vi "actuate_singleJumpExp_v0.04.vi"(0 "Phase Cluster":T2, 1 "valve Time Cluster":T1, 2 "Didn't Lift?":bool, 3 "data in":T3={"daq_ao 1"="Dev1/ao0", "daq_ai 1"="Dev1/ai0", "experiment day folder"=path "D:/DATA/8-27-15 save func testing/test.lvm", "Multiclamp init error"=0, "Multiclamp Handle Out"=0, "sampling rate (Hz)"=10000, "trial name"=""}, 5 "PhaseLetter":string, 7 "controls array in":refnum<vi>[](array[refnum]), 9 "time to wait for solution change (min)":dbl=2.5 min=0.0 step=0.01, 11 "error in":errorcluster, 12 "common cluster":T6, 13 "individual controls in":T5) -> (4 "output cluster":T4={"daq_ao 2"="", "Duration (s)"=0.0, "Sample Freq (Hz)"=0.0, "Phase"=0.0, "Duty Cycle"=0.0, "Jump Filter Freq (Hz)"=0.0, "Number of Replicates"=1} {"Number of Replicates" min=1 max=10}, 6 "protocol waveform":waveform(dbl)(graph), 8 "jumptestMonitor":waveform(dbl)[](graph) caption="protocol response", 10 "control array out":refnum<vi>[](array[refnum]), 14 "experiment VI ref":refnum<vi>, 15 "error out":errorcluster)   [LabVIEW 2019]
uses:
  pipette cleaning/pressure box/cleaning_soft/controls/actuator_type.ctl
  pipette cleaning/pressure box/cleaning_soft/controls/actuator_cluster.ctl
  machine_vision/coordinate model vis/transform_properties_actuators.ctl
  machine_vision/controls/transform_cluster_actuator.ctl
  controls/NH_method.ctl
  pipette cleaning/pressure box/cleaning_soft/controls/pressure_box_type.ctl
  pipette cleaning/pressure box/cleaning_soft/controls/pressure_box_control.ctl
  multipatch/controls/multipatch_common_controls_v4.ctl
  controls/memtest_def.ctl
  multipatch/controls/multipatch_individual_controls_v5.ctl
  Controls/Data.ctl
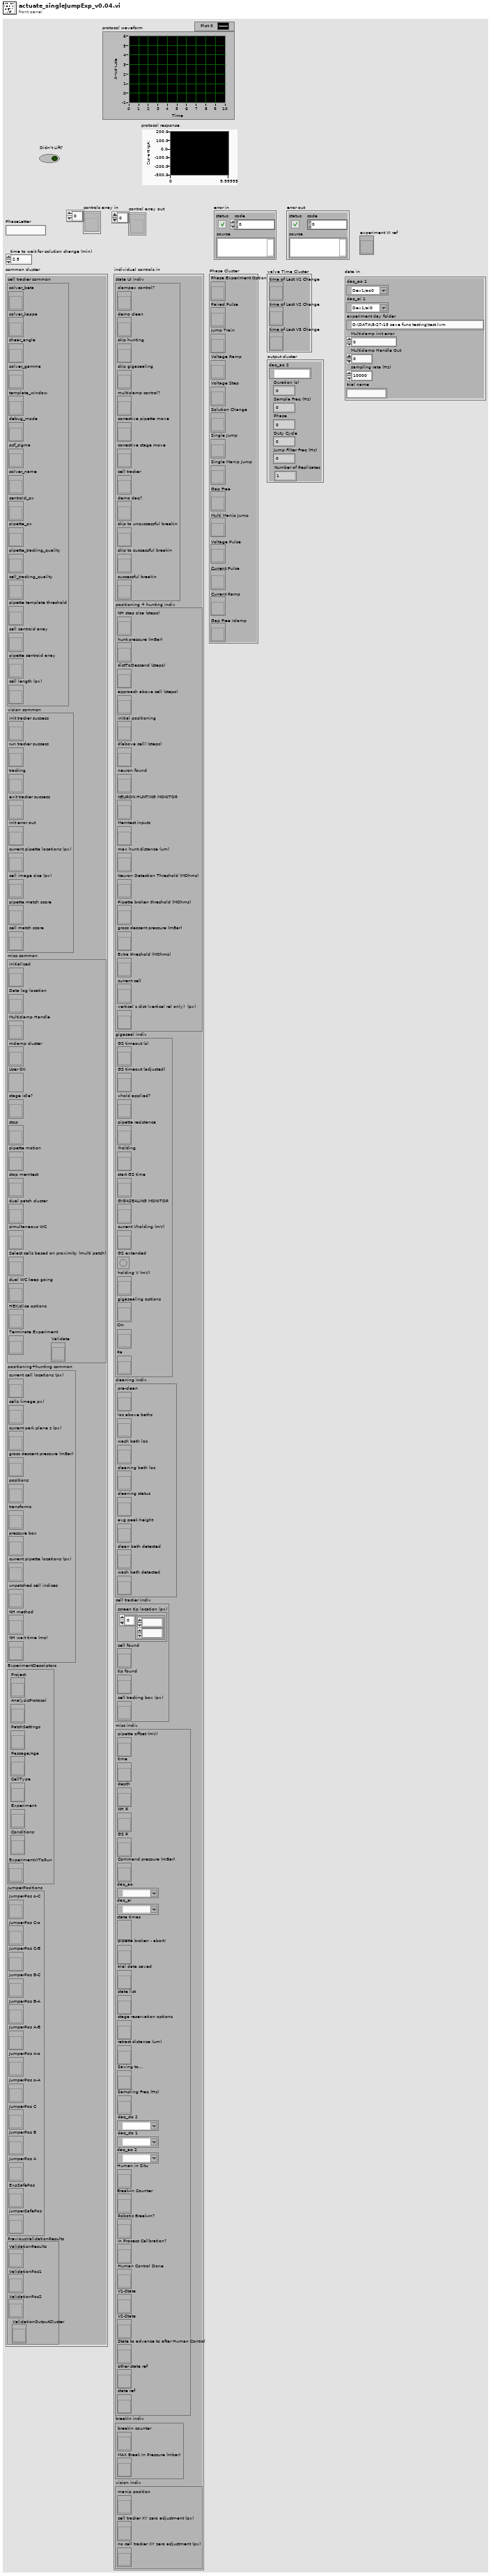
[diagram p1: front panel]
types:
  T1 = cluster{"time of Last V1 Change":refnum<vi>, "time of Last V2 Change":refnum<vi>, "time of Last V3 Change":refnum<vi>}
  T2 = cluster{"Phase Experiment Option":refnum<vi>, "Paired Pulse":refnum<vi>, "Jump Train":refnum<vi>, "Voltage Ramp":refnum<vi>, "Voltage Step":refnum<vi>, "Solution Change":refnum<vi>, "Single Jump":refnum<vi>, "Single Manip Jump":refnum<vi>, "Gap Free":refnum<vi>, "Multi Manip Jump":refnum<vi>, "Voltage Pulse":refnum<vi>, "Current Pulse":refnum<vi>, "Current Ramp":refnum<vi>, "Gap Free Iclamp":refnum<vi>}
  T3 = typedef "Data.ctl" = cluster{"daq_ao 1":tag, "daq_ai 1":tag, "experiment day folder":path, "Multiclamp init error":i32, "Multiclamp Handle Out":u32, "sampling rate (Hz)":i32, "trial name":string}
  T4 = cluster{"daq_ao 2":tag, "Duration (s)":dbl, "Sample Freq (Hz)":dbl, "Phase":dbl, "Duty Cycle":dbl, "Jump Filter Freq (Hz)":dbl, "Number of Replicates":i16}
  T5 = typedef "multipatch_individual_controls_v5.ctl" = cluster{"state UI indiv":cluster{"clampex control?":refnum<vi>, "demo clean":refnum<vi>, "skip hunting":refnum<vi>, "skip gigasealing":refnum<vi>, "multiclamp control?":refnum<vi>, "corrective pipette move":refnum<vi>, "corrective stage move":refnum<vi>, "cell tracker":refnum<vi>, "demo daq?":refnum<vi>, "skip to unsuccessful breakin":refnum<vi>, "skip to successful breakin":refnum<vi>, "successful breakin":refnum<vi>}, "positioning + hunting indiv":cluster{"NH step size (steps)":refnum<vi>, "hunt pressure (mBar)":refnum<vi>, "distToDescend (steps)":refnum<vi>, "approach above cell (steps)":refnum<vi>, "initial positioning":refnum<vi>, "d(above cell) (steps)":refnum<vi>, "neuron found":refnum<vi>, "NEURON HUNTING MONITOR":refnum<vi>, "Memtest inputs":refnum<vi>, "max hunt distance (um)":refnum<vi>, "Neuron Detection Threshold (MOhms)":refnum<vi>, "Pipette broken threshold (MOhms)":refnum<vi>, "gross descent pressure (mBar)":refnum<vi>, "Extra threshold (MOhms)":refnum<vi>, "current cell":refnum<vi>, "vertical z dist (vertical rel only)  (px)":refnum<vi>}, "gigaseal indiv":cluster{"GS timeout (s)":refnum<vi>, "GS timeout (adjusted)":refnum<vi>, "vhold applied?":refnum<vi>, "pipette resistance":refnum<vi>, "Iholding":refnum<vi>, "start GS time":refnum<vi>, "GIGASEALING MONITOR":refnum<vi>, "current Vholding (mV)":refnum<vi>, "GS extended":refnum<vi>, "holding V (mV)":refnum<vi>, "gigasealing options":refnum<vi>, "Cm":refnum<vi>, "Ra ":refnum<vi>}, "cleaning indiv":cluster{"pre-clean":refnum<vi>, "loc above baths":refnum<vi>, "wash bath loc":refnum<vi>, "cleaning bath loc":refnum<vi>, "cleaning status":refnum<vi>, "avg peak height":refnum<vi>, "clean bath detected":refnum<vi>, "wash bath detected":refnum<vi>}, "cell tracker indiv":cluster{"screen tip location (px)":refnum<vi>, "cell found":refnum<vi>, "tip found":refnum<vi>, "cell tracking box (px)":refnum<vi>}, "misc indiv":cluster{"pipette offset (mV)":refnum<vi>, "time":refnum<vi>, "depth":refnum<vi>, "NH R":refnum<vi>, "GS R":refnum<vi>, "Command pressure (mBar)":refnum<vi>, "daq_ao":tag, "daq_ai":tag, "state times":refnum<vi>, "pipette broken - abort!":refnum<vi>, "trial data saved":refnum<vi>, "state list":refnum<vi>, "stage reservation options":refnum<vi>, "retract distance (um)":refnum<vi>, "Saving to...":refnum<vi>, "Sampling Freq (Hz)":refnum<vi>, "daq_do 2":tag, "daq_do 1":tag, "daq_ao 2":tag, "Human in Situ":refnum<vi>, "Break-In Counter":refnum<vi>, "Robotic Break-In?":refnum<vi>, "In Process Calibration?":refnum<vi>, "Human Control Done":refnum<vi>, "V1-State":refnum<vi>, "V2-State":refnum<vi>, "State to advance to after Human Control":refnum<vi>, "other state ref":refnum<vi>, "state ref":refnum<vi>}, "breakin indiv":cluster{"breakin counter":refnum<vi>, "MAX Break In Pressure (mbar)":refnum<vi>}, "vision indiv":cluster{"manip position":refnum<vi>, "cell tracker XY zero adjustment (px)":refnum<vi>, "no cell tracker XY zero adjustment (px)":refnum<vi>}}
  T6 = typedef "multipatch_common_controls_v4.ctl" = cluster{"cell tracker common":cluster{"solver_beta":refnum<vi>, "solver_kappa":refnum<vi>, "shear_angle":refnum<vi>, "solver_gamma":refnum<vi>, "template_window":refnum<vi>, "debug_mode":refnum<vi>, "psf_sigma":refnum<vi>, "solver_name":refnum<vi>, "centroid_px":refnum<vi>, "pipette_px":refnum<vi>, "pipette_tracking_quality":refnum<vi>, "cell_tracking_quality":refnum<vi>, "pipette template threshold":refnum<vi>, "cell centroid array":refnum<vi>, "pipette centroid array":refnum<vi>, "cell length (px)":refnum<vi>}, "vision common":cluster{"init tracker success":refnum<vi>, "run tracker success":refnum<vi>, "tracking":refnum<vi>, "exit tracker success":refnum<vi>, "init error out":refnum<vi>, "current pipette locations (px)":refnum<vi>, "cell image size (px)":refnum<vi>, "pipette match score":refnum<vi>, "cell match score":refnum<vi>}, "misc common":cluster{"initialized":refnum<vi>, "Data log location":refnum<vi>, "Multiclamp Handle":refnum<vi>, "mclamp cluster":refnum<vi>, "User OK":refnum<vi>, "stage idle?":refnum<vi>, "stop":refnum<vi>, "pipette motion":refnum<vi>, "stop memtest":refnum<vi>, "dual patch cluster":refnum<vi>, "simultaneous WC":refnum<vi>, "Select cells based on proximity (multi patch)":refnum<vi>, "dual WC keep going":refnum<vi>, "HEK/slice options":refnum<vi>, "Terminate Experiment":refnum<vi>, "Validate":refnum<vi>}, "positioning+hunting common":cluster{"current cell locations (px)":refnum<vi>, "cells (image px)":refnum<vi>, "current park plane z (px)":refnum<vi>, "gross descent pressure (mBar)":refnum<vi>, "positions":refnum<vi>, "transforms":refnum<vi>, "pressure box":refnum<vi>, "current pipette locations (px)":refnum<vi>, "unpatched cell indices":refnum<vi>, "NH method":refnum<vi>, "NH wait time (ms)":refnum<vi>}, "ExperimentDescriptors":cluster{"Project":refnum<vi>, "AnalysisProtocol":refnum<vi>, "PatchSettings":refnum<vi>, "Passage/Age":refnum<vi>, "CellType":refnum<vi>, "Experiment":refnum<vi>, "Conditions":refnum<vi>, "ExperimentVIToRun":refnum<vi>}, "JumperPositions":cluster{"JumperPos o-C":refnum<vi>, "JumperPos C-o":refnum<vi>, "JumperPos C-B":refnum<vi>, "JumperPos B-C":refnum<vi>, "JumperPos B-A":refnum<vi>, "JumperPos A-B":refnum<vi>, "JumperPos A-o":refnum<vi>, "JumperPos o-A":refnum<vi>, "JumperPos C":refnum<vi>, "JumperPos B":refnum<vi>, "JumperPos A":refnum<vi>, "ExpSafePos":refnum<vi>, "jumperSafePos":refnum<vi>}, "PreviousValidationResults":cluster{"ValidationResults":refnum<vi>, "ValidationPos1":refnum<vi>, "ValidationPos2":refnum<vi>, "ValidationOutputCluster":refnum<vi>}}
  T7 = cluster{"Which Position to use for Experiment":enum16{"Jumper Safe Position", "Experiment Safe Position", "Jumper Position A", "Jumper Position B", "Jumper Position C", "Jumper Position o-A", "Jumper Position A-o", "Jumper Position A-B", "Jumper Position B-A", "Jumper Position B-C", "Jumper Position C-B", "Jumper Position C-o", "Jumper Position o-C", "Don't Move"}, "Start Position (N)":string, "Jump Position (m)":string, "Duration (s)":dbl, "Delay (s)":dbl, "Pulse Width (s)":dbl, "Valve 1 Position":i16, "Valve 2 Position":i16, "Replicates":dbl, "Vholding (mV)":dbl, "Valve 3 Position":i16, "valve 1 used now?":bool, "valve 2 used now?":bool, "valve 3 used now? ":bool, "protocol Preview":waveform(dbl)[]}
  T8 = enum16{"Jumper Safe Position", "Experiment Safe Position", "Jumper Position A", "Jumper Position B", "Jumper Position C", "Jumper Position o-A", "Jumper Position A-o", "Jumper Position A-B", "Jumper Position B-A", "Jumper Position B-C", "Jumper Position C-B", "Jumper Position C-o", "Jumper Position o-C", "Don't Move"}
  T9 = enum16{"manipulator 1", "manipulator 2", "manipulator 3", "manipulator 4"}
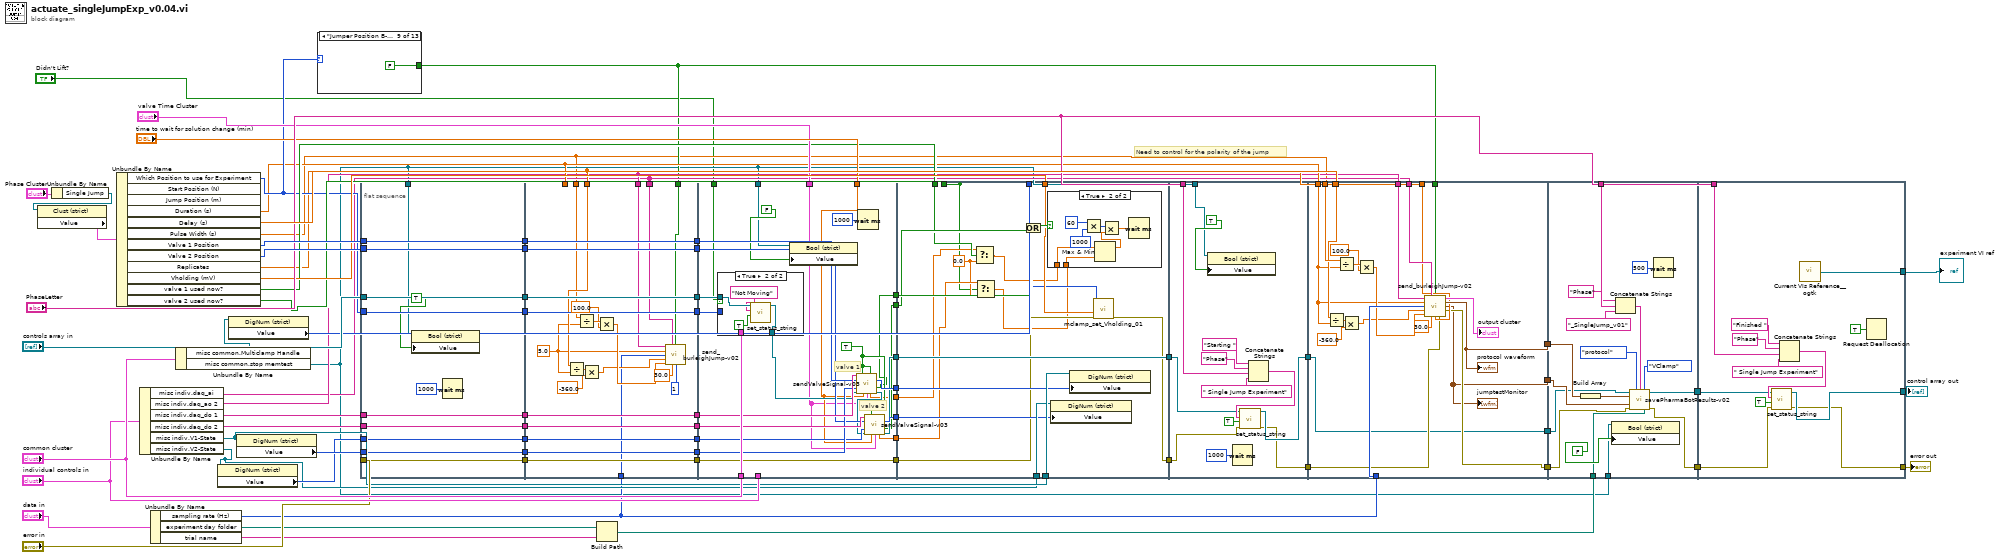
[diagram p0: block diagram]
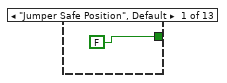
[diagram p2: hidden frame]
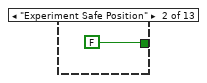
[diagram p3: hidden frame]
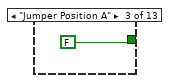
[diagram p4: hidden frame]
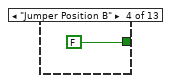
[diagram p5: hidden frame]
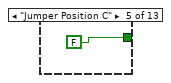
[diagram p6: hidden frame]
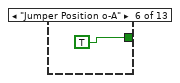
[diagram p7: hidden frame]
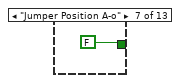
[diagram p8: hidden frame]
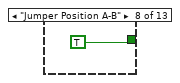
[diagram p9: hidden frame]
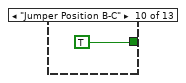
[diagram p10: hidden frame]
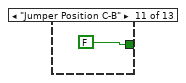
[diagram p11: hidden frame]
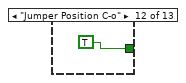
[diagram p12: hidden frame]
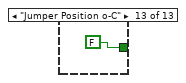
[diagram p13: hidden frame]
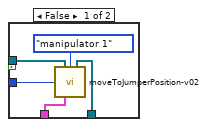
[diagram p14: hidden frame]
diagram:
  # "Need to control for the polarity of the jump"
  n1 = Unbundle By Name("Phase Cluster") -> ("Single Jump"=w55:refnum<vi>)
  n2 = property class="Clust (strict)"(reference=w55) -> ("Value"=w54:T7)  [unwired: 1 in, 2 out]
  n3 = Unbundle By Name(w54) -> ("Which Position to use for Experiment"=w29:T8, "Duration (s)"=w19:dbl, "Delay (s)"=w51:dbl, "Pulse Width (s)"=w3:dbl, "Valve 1 Position"=w53:i16, "Valve 2 Position"=w52:i16, "Replicates"=w18:dbl, "Vholding (mV)"=w38:dbl, "valve 1 used now?"=w31:bool, "valve 2 used now?"=w30:bool)  [unwired: 2 out]
  n4 = Unbundle By Name("individual controls in") -> ("misc indiv.daq_ai"=w15:tag, "misc indiv.daq_ao 2"=w16:tag, "misc indiv.daq_do 1"=w75:tag, "misc indiv.daq_do 2"=w74:tag, "misc indiv.V1-State"=w66:refnum<vi>, "misc indiv.V2-State"=w65:refnum<vi>)
  n5 = Unbundle By Name("data in") -> ("sampling rate (Hz)"=w17:i32, "experiment day folder"=w59:path, "trial name"=w58:string)
  n6 = Unbundle By Name("common cluster") -> ("misc common.Multiclamp Handle"=w37:refnum<vi>, "misc common.stop memtest"=w4:refnum<vi>)
  n7 = property class="DigNum (strict)"(reference=w65) -> ("Value"=w67:u16)  [unwired: 1 in, 2 out]
  n8 = property class="DigNum (strict)"(reference=w37) -> ("Value"=w36:u32)  [unwired: 1 in, 2 out]
  n9 = property class="DigNum (strict)"(reference=w66) -> ("Value"=w68:u16)  [unwired: 1 in, 2 out]
  n10 = case shown="\"Jumper Position B-A\"" w29 {
    tunnel: [FALSE FALSE FALSE FALSE FALSE TRUE FALSE TRUE FALSE TRUE FALSE TRUE FALSE] -> w14
    frame "Jumper Safe Position", Default {
    }
    frame "Experiment Safe Position" {
    }
    frame "Jumper Position A" {
    }
    frame "Jumper Position B" {
    }
    frame "Jumper Position C" {
    }
    frame "Jumper Position o-A" {
    }
    frame "Jumper Position A-o" {
    }
    frame "Jumper Position A-B" {
    }
    frame "Jumper Position B-A" {
    }
    frame "Jumper Position B-C" {
    }
    frame "Jumper Position C-B" {
    }
    frame "Jumper Position C-o" {
    }
    frame "Jumper Position o-C" {
    }
  }
  n11 = flat-sequence {
    tunnel: "controls array in" -> [w94]
    tunnel: w52 -> [w95]
    tunnel: w53 -> [w96]
    tunnel: w67 -> [w97]
    tunnel: w68 -> [w98]
    tunnel: "error in" -> [w99]
    tunnel: w74 -> [w100]
    tunnel: w75 -> [w101]
    tunnel: w29 -> [w102]
    tunnel: [w102] -> w13
    tunnel: [w101] -> w12
    tunnel: [w100] -> w11
    tunnel: [w99] -> w10
    tunnel: [w98] -> w9
    tunnel: [w97] -> w8
    tunnel: [w96] -> w7
    tunnel: [w95] -> w6
    tunnel: [w94] -> w5
    tunnel: w4 -> [w92]
    tunnel: [w126] -> w28
    tunnel: [w125] -> w27
    tunnel: [w124] -> w26
    tunnel: [w123] -> w25
    tunnel: [w122] -> w24
    tunnel: [w121] -> w23
    tunnel: [w120] -> w22
    tunnel: [w119] -> w21
    tunnel: [w118] -> w20
    tunnel: w19 -> [_]
    tunnel: w18 -> [w111]
    tunnel: w3 -> [w110]
    tunnel: w17 -> [w109]
    tunnel: w16 -> [w108]
    tunnel: w15 -> [w107]
    tunnel: w14 -> [w105]
    tunnel: w13 -> [w126]
    tunnel: w12 -> [w125]
    tunnel: w11 -> [w124]
    tunnel: w10 -> [w123]
    tunnel: w9 -> [w122]
    tunnel: w8 -> [w121]
    tunnel: w7 -> [w120]
    tunnel: w6 -> [w119]
    tunnel: w5 -> [w118]
    tunnel: "common cluster" -> [w151]
    tunnel: "individual controls in" -> [_]
    tunnel: [w148] -> w70
    tunnel: [w145] -> w64
    tunnel: [w144] -> w63
    tunnel: [w138] -> w45
    tunnel: [w136] -> w40
    tunnel: [w135] -> w39
    tunnel: "time to wait for solution change (min)" -> [w134]
    tunnel: "valve Time Cluster" -> [w133]
    tunnel: [w132] -> w33
    tunnel: [w131] -> w32
    tunnel: w28 -> [w152]
    tunnel: w27 -> [w150]
    tunnel: w26 -> [w149]
    tunnel: w25 -> [w148]
    tunnel: w24 -> [w147]
    tunnel: w23 -> [w146]
    tunnel: w22 -> [w143]
    tunnel: w21 -> [w142]
    tunnel: w20 -> [w141]
    tunnel: w4 -> [w129]
    tunnel: "Didn't Lift?" -> [w127]
    tunnel: [w169] -> w71
    tunnel: w70 -> [w171]
    tunnel: w66 -> [w180]
    tunnel: w65 -> [w179]
    tunnel: w64 -> [w178]
    tunnel: w63 -> [w177]
    tunnel: [w176] -> w46
    tunnel: w45 -> [w176]
    tunnel: w40 -> [w174]
    tunnel: w39 -> [w173]
    tunnel: w38 -> [w172]
    tunnel: w36 -> [w170]
    tunnel: w33 -> [w166]
    tunnel: w32 -> [w165]
    tunnel: w31 -> [w167]
    tunnel: [w162] -> _
    tunnel: w30 -> [w162]
    tunnel: w4 -> [w188]
    tunnel: [w190] -> w72
    tunnel: w71 -> [w191]
    tunnel: [w192] -> w47
    tunnel: w46 -> [w193]
    tunnel: "PhaseLetter" -> [w194]
    tunnel: w15 -> [w220]
    tunnel: w16 -> [w219]
    tunnel: w72 -> [w205]
    tunnel: [w217] -> w62
    tunnel: [w202] -> w61
    tunnel: w18 -> [w207]
    tunnel: w19 -> [w206]
    tunnel: w17 -> [w216]
    tunnel: w3 -> [w214]
    tunnel: w51 -> [w211]
    tunnel: [w204] -> w50
    tunnel: [w203] -> w48
    tunnel: w47 -> [w203]
    tunnel: w14 -> [w201]
    tunnel: w4 -> [w237]
    tunnel: w62 -> [w236]
    tunnel: w61 -> [w234]
    tunnel: w57 -> [w231]
    tunnel: "PhaseLetter" -> [w229]
    tunnel: w50 -> [w226]
    tunnel: w48 -> [w225]
    tunnel: [w223] -> w43
    tunnel: [w224] -> w42
    tunnel: [w244] -> w44
    tunnel: [w243] -> w69
    tunnel: w43 -> [w242]
    tunnel: w42 -> [w245]
    tunnel: "PhaseLetter" -> [w241]
    tunnel: [w240] -> w1
    frame #0 {
      n12 = property class="Bool (strict)"(reference=w92, "Value"=TRUE ("stop memtest")) -> ()  [unwired: 1 in, 2 out]
      n13 = Wait (ms)(milliseconds to wait=u32 1000) -> ()  [unwired: 1 out]
    }
    frame #1 {
      w103 = 5.0 ("y")
      n14 = Divide(x=w111, y=w103) -> (x/y=w113:dbl)
      n15 = Divide(x=w110, y=w103) -> (x/y=w116:dbl)
      n16 = Multiply(x=w113, y=-360.0) -> (x*y=w112:dbl)
      n17 = Multiply(x=w116, y=100.0) -> (x*y=w114:dbl)
      n18 = call "send_burleighJump-v02.vi"("daq_ao 2"=w108, "daq_ai"=w107, "Jump Polarity"=w105, "Duration (s)"=w103, "Sample Freq (Hz)"=w109, "Phase"=w112, "Duty Cycle"=w114, "Jump Filter Freq (Hz)"=30.0, "Number of Replicates"=i16 1) -> ()  [unwired: 3 in, 4 out]
    }
    frame #2 {
      w137 = TRUE ("Set Status")
      # "valve 2"
      # "valve 1"
      n19 = case shown="True" w127 {
        tunnel: w152 -> [w157 _]
        tunnel: w151 -> [w156 _]
        tunnel: w141 -> [w154 w160]
        tunnel: [w153 w159] -> w140
        frame False {
          n20 = call "moveToJumperPosition-v02.vi"("which manipulator"=T9."manipulator 1", "controls array in"=w154, "Which Jumper Position to move to?"=w157, "common cluster"=w156) -> ("control array out"=w153:refnum<vi>[])  [unwired: 10 in, 1 out]
        }
        frame True {
          n21 = call "set_status_string.vi"("new line?"=TRUE, "status string in"="Not Moving", "controls array"=w160) -> ("controls array out"=w159:refnum<vi>[])  [unwired: 7 in, 1 out]
        }
      }
      n22 = property class="Bool (strict)"(reference=w129, "Value"=FALSE ("stop memtest")) -> ()  [unwired: 1 in, 2 out]
      n23 = call "sendValveSignal-v03.vi"("daq_do"=w150, "Set Status"=w137, "Valve1?"=w137, "ChangeToValve"=w143, "CurrentValve"=w147, "controls array in"=w140, "time to wait for solution change (min)"=w134, "valve Time Cluster"=w133) -> ("ValveSetTo"=w144:u16, "valve changed?"=w136:bool, "additional time to wait (min)"=w132:dbl, "control array out"=w139:refnum<vi>[])  [unwired: 4 in]
      n24 = Wait (ms)(milliseconds to wait=u32 1000) -> ()  [unwired: 1 out]
      n25 = call "sendValveSignal-v03.vi"("daq_do"=w149, "Set Status"=w137, "ChangeToValve"=w142, "CurrentValve"=w146, "controls array in"=w139, "time to wait for solution change (min)"=w134, "valve Time Cluster"=w133) -> ("ValveSetTo"=w145:u16, "valve changed?"=w135:bool, "additional time to wait (min)"=w131:dbl, "control array out"=w138:refnum<vi>[])  [unwired: 5 in]
    }
    frame #3 {
      w163 = 0.0 ("f")
      n26 = Select(t=w166, s=w167, f=w163) -> (s? t:f=w168:dbl)
      n27 = Select(t=w165, s=w162, f=w163) -> (s? t:f=w164:dbl)
      n28 = Or(x=w174, y=w173) -> (x .or. y?=w175:bool)
      n29 = case shown="True" w175 {
        tunnel: w168 -> [_ w183]
        tunnel: w164 -> [_ w182]
        frame False {
        }
        frame True {
          n30 = Multiply(x=u32 60 ("milliseconds to wait"), y=u32 1000) -> (x*y=w185:u32)
          n31 = Max & Min(x=w183, y=w182) -> (max(x,y)=w181:dbl)  [unwired: 1 out]
          n32 = Multiply(x=w185, y=w181) -> (x*y=w184:dbl)
          n33 = Wait (ms)(milliseconds to wait=w184) -> ()  [unwired: 1 out]
        }
      }
      n34 = property class="DigNum (strict)"(reference=w179, "Value"=w178) -> ()  [unwired: 1 in, 2 out]
      n35 = property class="DigNum (strict)"(reference=w180, "Value"=w177) -> ()  [unwired: 1 in, 2 out]
      n36 = call "mclamp_set_Vholding_01.vi"("error in (no error)"=w171, "set holding (mV)"=w172, "Multiclamp Handle Out"=w170) -> ("error out"=w169:errorcluster)  [unwired: 7 in, 1 out]
    }
    frame #4 {
      n37 = property class="Bool (strict)"(reference=w188, "Value"=TRUE ("stop memtest")) -> ()  [unwired: 1 in, 2 out]
      n38 = Wait (ms)(milliseconds to wait=u32 1000) -> ()  [unwired: 1 out]
      n39 = Concatenate Strings("Starting " ("string"), "Phase" ("string"), w194, " Single Jump Experiment" ("string")) -> (w196:string)
      n40 = call "set_status_string.vi"("error in"=w191, "new line?"=TRUE, "status string in"=w196, "controls array"=w193) -> ("error out"=w190:errorcluster, "controls array out"=w192:refnum<vi>[])  [unwired: 6 in]
    }
    frame #5 {
      n41 = Divide(x=w211, y=w206) -> (x/y=w209:dbl)
      n42 = Divide(x=w214, y=w206) -> (x/y=w215:dbl)
      n43 = Multiply(x=w209, y=-360.0) -> (x*y=w208:dbl)
      n44 = Multiply(x=w215, y=100.0) -> (x*y=w212:dbl)
      n45 = call "send_burleighJump-v02.vi"("daq_ao 2"=w219, "daq_ai"=w220, "Jump Polarity"=w201, "Duration (s)"=w206, "Sample Freq (Hz)"=w216, "Phase"=w208, "Duty Cycle"=w212, "Jump Filter Freq (Hz)"=30.0, "Number of Replicates"=w207, "error in"=w205) -> ("output cluster"=→"output cluster":T4, "output waveform"=w217:waveform(dbl), "protocol response"=w202:waveform(dbl)[], "error out"=w204:errorcluster)  [unwired: 2 in]
      "jumptestMonitor" <- w202
      "protocol waveform" <- w217
    }
    frame #6 {
      n46 = Build Array(w236) -> (w235:waveform(dbl)[])
      n47 = property class="Bool (strict)"(reference=w237, "Value"=FALSE ("stop memtest")) -> ()  [unwired: 1 in, 2 out]
      n48 = Concatenate Strings("Phase" ("string"), w229, "_SingleJump_v01" ("string")) -> (w230:string)
      n49 = call "savePharmaBotResults-v02.vi"("controls array"=w225, "protocol or memtest"=enum16{"protocol", "memtest", "validation"}."protocol", "ExpPhase"=w230, "which clamp"=enum16{"VClamp", "IClamp"}."VClamp", "protocol waveform"=w235, "protocol response"=w234, "error in"=w226, "Save to (folder dir)"=w231) -> ("controls array out"=w224:refnum<vi>[], "error out"=w223:errorcluster)  [unwired: 6 in]
      n50 = Wait (ms)(milliseconds to wait=u32 500) -> ()  [unwired: 1 out]
    }
    frame #7 {
      n51 = Concatenate Strings("Finished " ("string"), "Phase" ("string"), w241, " Single Jump Experiment" ("string")) -> (w247:string)
      n52 = call "set_status_string.vi"("error in"=w242, "new line?"=TRUE, "status string in"=w247, "controls array"=w245) -> ("error out"=w243:errorcluster, "controls array out"=w244:refnum<vi>[])  [unwired: 6 in]
      n53 = call "Current VIs Reference__ogtk.vi"() -> ("Current VI's reference"=w240:refnum<vi>)  [unwired: 5 in]
      n54 = Request Deallocation(TRUE ("flag")) -> ()
    }
  }
  n55 = Build Path(base path=w59, name or relative path=w58) -> (appended path=w57:path)
  "error out" <- w69
  "control array out" <- w44
  "experiment VI ref" <- w1
